vi "fgv_4610_visa.vi"(7 "cmd":T1, 8 "error in":errorcluster) -> (0 "error out":errorcluster)   [LabVIEW 2019]
uses:
  _ctrl/BP4610_cmd.ctl
  _ctrl/init-r-stop.ctl
  SubVIs/common/cmd_err.ctl
  _ctrl/rw.ctl
  Type def/SetNF_BP4610.ctl
  SubVIs/common/Glob_Ref.vi
panel:
  out "OverLoad":i32 caption="Query"
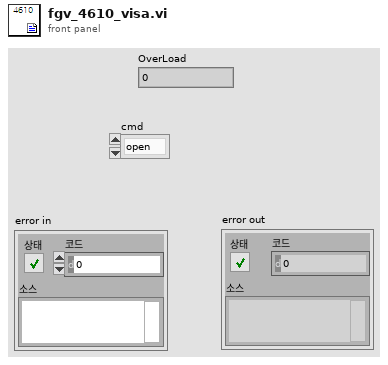
[diagram p1: front panel]
types:
  T1 = typedef "BP4610_cmd.ctl" = enum16{"open", "read", "set", "set_seq", "limit", "limit_seq", "output on", "output off", "close"}
  T2 = enum16{"DL950", "BP4610", "DSP1500", "cDAQ-AI", "cDAQ-AO", "cDAQ-DO"}
  T3 = typedef "init-r-stop.ctl" = enum16{"ini", "read", "stop"}
  T4 = typedef "cmd_err.ctl" = enum16{"close", "open", "default"}
  T5 = typedef "rw.ctl" = enum16{"read", "write"}
  T6 = typedef "SetNF_BP4610.ctl" = cluster{"Set":enum16{"Current", "Voltage", "FREQ/WAVE"}, "Operation mode":u16, "Voltage[Vp-p]":dbl, "Current[Ap-p]":dbl, "Voltage[V]":dbl, "Current[A]":dbl, "Frequency[Hz]":dbl, "Waveform":enum16{"Sine", "Square", "ARB 1", "ARB 2", "ARB 3", "ARB 4", "ARB 5", "ARB 6", "ARB 7", "ARB 8", "ARB 9", "ARB 10", "ARB 11", "ARB 12", "ARB 13", "ARB 14", "ARB 15", "ARB 16"}}
  T7 = typedef "BP4610_config.ctl" = cluster{"VISA":refnum<visa-resource-name>, "Limit-BP":cluster{"Set":enum16{"Current", "Voltage"}, "Voltage+[V]":dbl, "Current+[A]":dbl, "Voltage-[V]":dbl, "Current-[A]":dbl}, "SET BP":cluster{"Set":enum16{"Current", "Voltage", "FREQ/WAVE"}, "Operation mode":u16, "Voltage[Vp-p]":dbl, "Current[Ap-p]":dbl, "Voltage[V]":dbl, "Current[A]":dbl, "Frequency[Hz]":dbl, "Waveform":enum16{"Sine", "Square", "ARB 1", "ARB 2", "ARB 3", "ARB 4", "ARB 5", "ARB 6", "ARB 7", "ARB 8", "ARB 9", "ARB 10", "ARB 11", "ARB 12", "ARB 13", "ARB 14", "ARB 15", "ARB 16"}}}
  T8 = typedef "BP4610_return.ctl" = cluster{"DC voltage[V]":dbl, "DC current[A]":dbl}
  T9 = cluster{"Set":enum16{"Current", "Voltage", "FREQ/WAVE"}, "Operation mode":u16, "Voltage[Vp-p]":dbl, "Current[Ap-p]":dbl, "Voltage[V]":dbl, "Current[A]":dbl, "Frequency[Hz]":dbl, "Waveform":enum16{"Sine", "Square", "ARB 1", "ARB 2", "ARB 3", "ARB 4", "ARB 5", "ARB 6", "ARB 7", "ARB 8", "ARB 9", "ARB 10", "ARB 11", "ARB 12", "ARB 13", "ARB 14", "ARB 15", "ARB 16"}}
  T10 = typedef "cap_config.ctl" = cluster{"Test Mode":enum32{"6.3.2 저온 작동/방치 시험", "6.3.3 고온 작동/방치 시험", "6.3.4 온도 싸이클 시험", "6.3.6 온습도 싸이클 시험", "6.3.8 결로 시험", "6.3.9 빙결 시험", "ON/OFF 동작시험"}, "ON time[ms]":dbl, "OFF time[ms]":dbl, "1. 작동시간[분]":dbl, "2. 미작동시간[분]":dbl, "3. 작동시간[분]":dbl, "level[V]":dbl, "duty":dbl, "Freq":dbl, "Voltage+[V]":dbl, "Voltage-[V]":dbl, "Current+[A]":dbl, "Current-[A]":dbl, "출력전압[V]":dbl, "출력전류[A]":dbl, "OVP Level":dbl, "OCP Level":dbl, "Time Div":u16, "Record Len":i32, "방전 기준[V]":dbl, "Repeate (Each Ch)":u32, "Cycle[N]":u32, "ON/OFF 회 수[N]":dbl, "TrigPos[%]":dbl, "시험시간[분]":dbl}
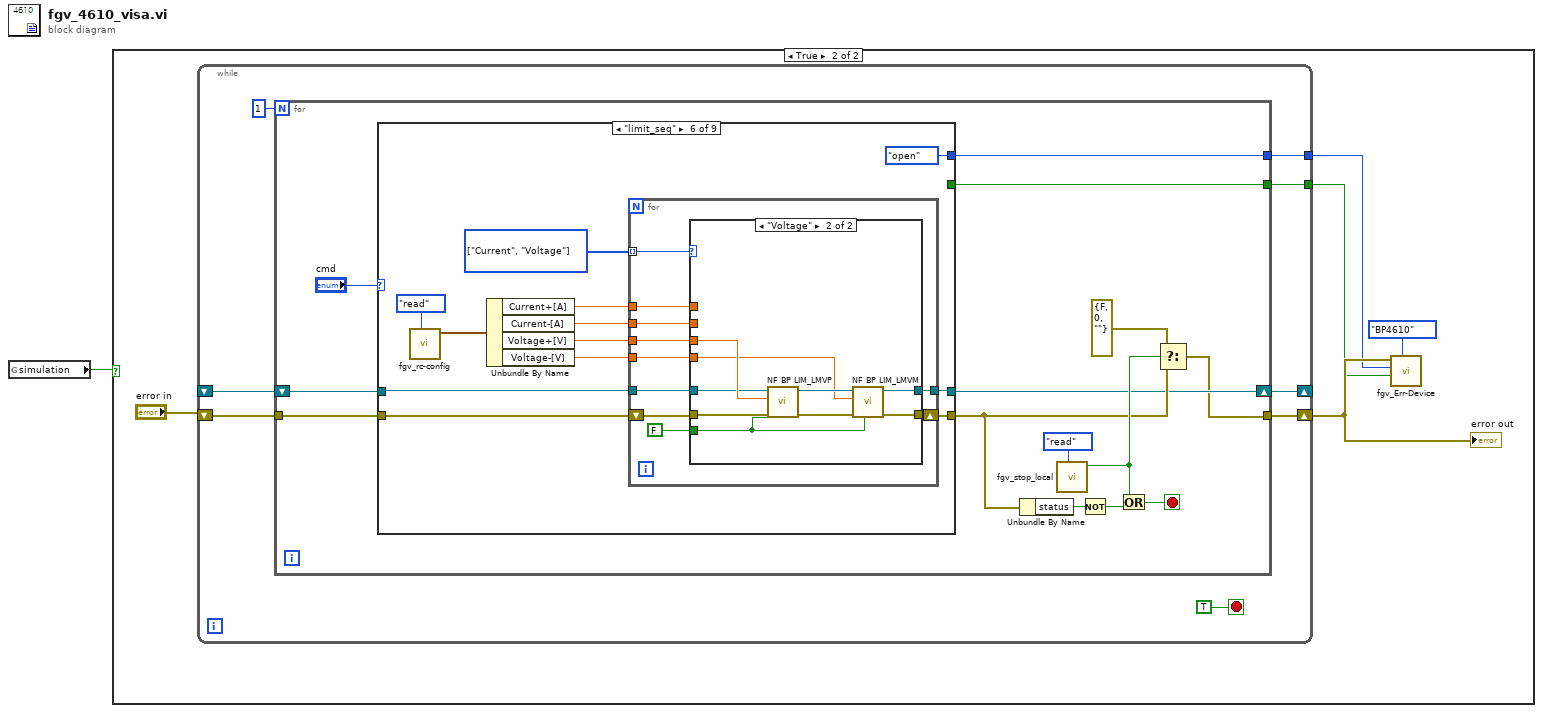
[diagram p0: block diagram]
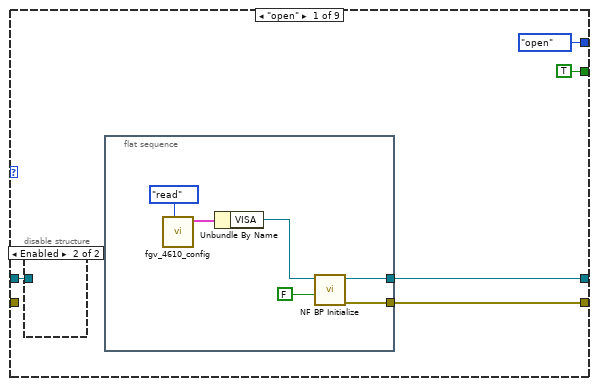
[diagram p3: hidden frame]
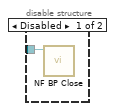
[diagram p4: hidden frame]
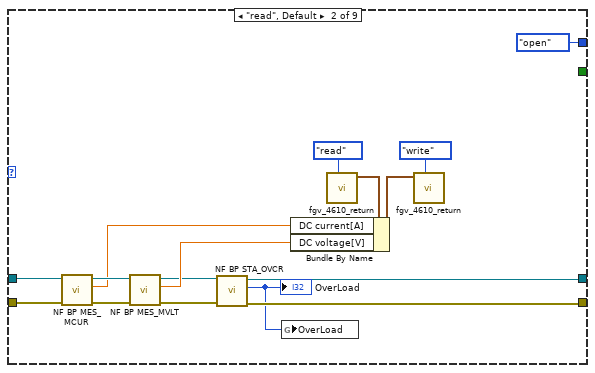
[diagram p5: hidden frame]
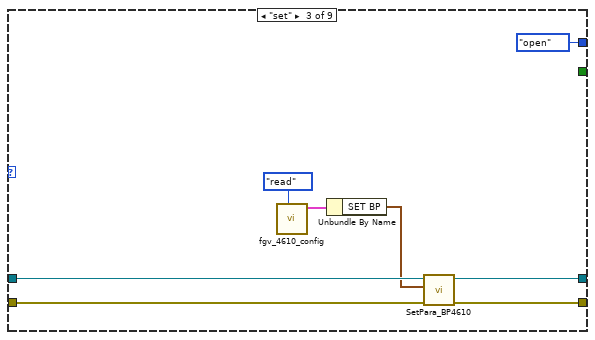
[diagram p6: hidden frame]
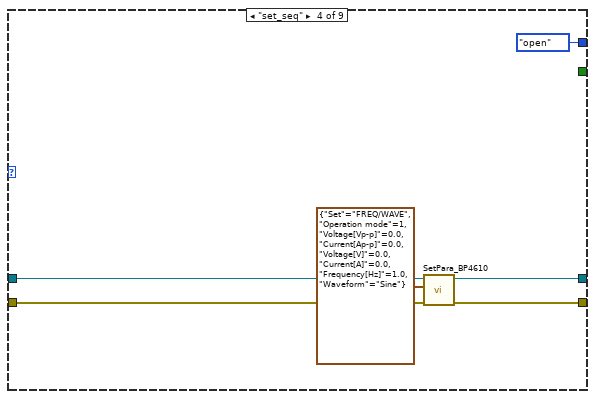
[diagram p7: hidden frame]
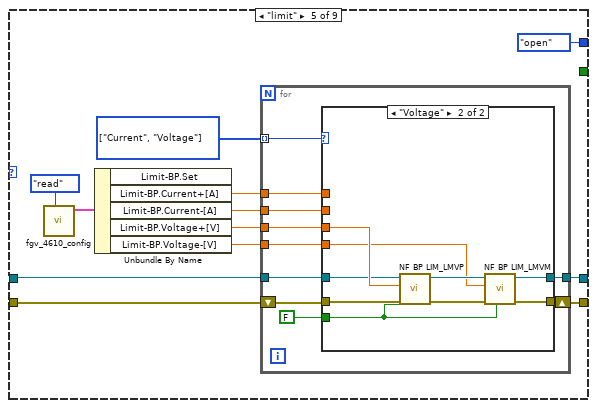
[diagram p8: hidden frame]
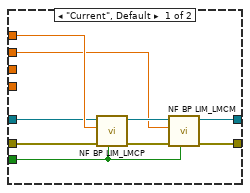
[diagram p9: hidden frame]
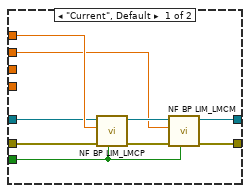
[diagram p10: hidden frame]
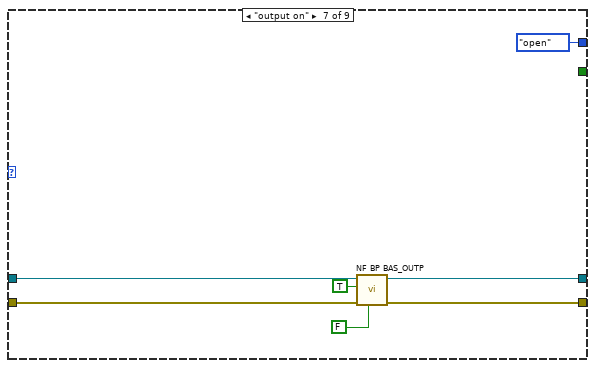
[diagram p11: hidden frame]
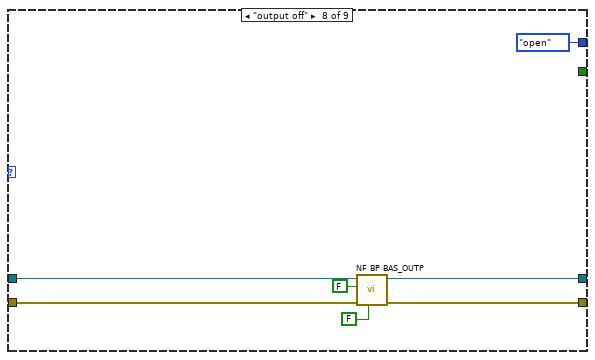
[diagram p12: hidden frame]
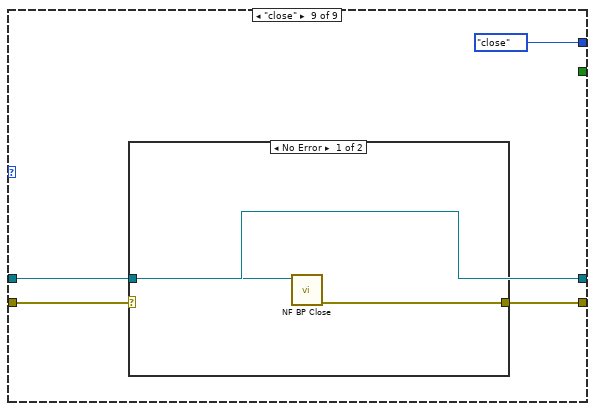
[diagram p13: hidden frame]
diagram:
  n1 = global read "Glob_Ref.vi" "simulation"() -> (w1:bool)
  n2 = case shown="True" w1 {
    frame False {
    }
    frame True {
      n3 = while {
        shift-right: [w11] -> _
        shift-left: _ -> [w13]
        shift-right: [w12] -> w5
        shift-left: "error in" -> [w9]
        tunnel: [w8] -> w4
        tunnel: [w7] -> w3
        stop <- TRUE stop-if-true
        n4 = for {
          N: 1 -> [_]
          tunnel: [w15] -> w12
          shift-right: [w16] -> w11
          shift-left: w13 -> [w27]
          tunnel: w9 -> [w19]
          tunnel: [w18] -> w8
          tunnel: [w17] -> w7
          stop <- w20 stop-if-true
          n5 = case shown="\"limit_seq\"" "cmd" {
            tunnel: [w33 w43 w64 w70 w80 w120 w153 w160 w166] -> w21
            tunnel: [w32 w44 w63 w69 w79 w119 w154 w161 w168] -> w16
            tunnel: w19 -> [_ w54 w61 w67 w81 w121 w155 w162 w167]
            tunnel: w27 -> [w31 w53 w62 w68 w82 w122 w156 w163 w168]
            tunnel: [cmd_err."open" ("cmd") cmd_err."open" ("cmd") cmd_err."open" ("cmd") cmd_err."open" ("cmd") cmd_err."open" ("cmd") cmd_err."open" ("cmd") cmd_err."open" ("cmd") cmd_err."open" ("cmd") cmd_err."close" ("cmd")] -> w18
            tunnel: [TRUE ("first?") _ _ _ _ _ _ _ _] -> w17
            frame "open" {
              n6 = disable-structure shown="Enabled" {
                disable-tunnel: w31 -> [w34 _]
                frame Disabled {
                  n7 = call <instrlib>:"NF BP Close.vi"("VISAsession"=w34) -> ()  [unwired: 10 in, 1 out]
                }
                frame Enabled {
                }
              }
              n8 = flat-sequence {
                tunnel: [w39] -> w33
                tunnel: [w38] -> w32
                frame #0 {
                  n9 = call "fgv_4610_config.vi"("cmd"=rw."read") -> ("BP4610 Config 2"=w36:T7)  [unwired: 9 in, 1 out]
                  n10 = Unbundle By Name(w36) -> ("VISA"=w35:refnum<visa-resource-name>)
                  n11 = call <instrlib>:"NF BP Initialize.vi"("Reset(T)"=FALSE ("Read"), "VISAsession"=w35) -> ("error out"=w39:errorcluster, "CopyVISAsession"=w38:refnum<visa-resource-name>)  [unwired: 7 in, 1 out]
                }
              }
            }
            frame "read", Default {
              n12 = call <instrlib>:"NF BP MES_MCUR.vi"("error in (no error)"=w54, "VISAsession"=w53) -> ("error out"=w56:errorcluster, "Query[A]"=w51:dbl, "CopyVISAsession"=w55:refnum<visa-resource-name>)  [unwired: 5 in, 2 out]
              n13 = call <instrlib>:"NF BP MES_MVLT.vi"("error in (no error)"=w56, "VISAsession"=w55) -> ("error out"=w45:errorcluster, "Query[V]"=w50:dbl, "CopyVISAsession"=w46:refnum<visa-resource-name>)  [unwired: 5 in, 2 out]
              n14 = call <instrlib>:"NF BP STA_OVCR.vi"("error in (no error)"=w45, "VISAsession"=w46) -> ("error out"=w43:errorcluster, "Query"=w42:i32, "CopyVISAsession"=w44:refnum<visa-resource-name>)  [unwired: 6 in, 1 out]
              "OverLoad" <- w42
              n15 = global write "Glob_Ref.vi" "OverLoad"(w42) -> ()
              n16 = call "fgv_4610_return.vi"("cmd"=rw."read") -> ("output 2"=w47:T8)  [unwired: 10 in]
              n17 = Bundle By Name(cluster=w47, "DC current[A]"=w51, "DC voltage[V]"=w50) -> (w49:T8)
              n18 = call "fgv_4610_return.vi"("cmd"=rw."write", "output"=w49) -> ()  [unwired: 9 in, 1 out]
            }
            frame "set" {
              n19 = call "fgv_4610_config.vi"("cmd"=rw."read") -> ("BP4610 Config 2"=w59:T7)  [unwired: 9 in, 1 out]
              n20 = Unbundle By Name(w59) -> ("SET BP"=w58:T9)
              n21 = call "SetPara_BP4610.vi"("error in"=w61, "SetBP"=w58, "VISA"=w62) -> ("error out"=w64:errorcluster, "VISA out"=w63:refnum<visa-resource-name>)  [unwired: 7 in]
            }
            frame "set_seq" {
              n22 = call "SetPara_BP4610.vi"("error in"=w67, "SetBP"=T6 {"Set"=enum."FREQ/WAVE", "Operation mode"=1, "Voltage[Vp-p]"=0.0, "Current[Ap-p]"=0.0, "Voltage[V]"=0.0, "Current[A]"=0.0, "Frequency[Hz]"=1.0, "Waveform"=enum."Sine"}, "VISA"=w68) -> ("error out"=w70:errorcluster, "VISA out"=w69:refnum<visa-resource-name>)  [unwired: 7 in]
            }
            frame "limit" {
              w72 = enum16{"Current", "Voltage"}[] [enum."Current", enum."Voltage"] items=["Current", "Voltage"]
              n23 = call "fgv_4610_config.vi"("cmd"=rw."read") -> ("BP4610 Config 2"=w77:T7)  [unwired: 9 in, 1 out]
              n24 = Unbundle By Name(w77) -> ("Limit-BP.Current+[A]"=w76:dbl, "Limit-BP.Current-[A]"=w75:dbl, "Limit-BP.Voltage+[V]"=w74:dbl, "Limit-BP.Voltage-[V]"=w73:dbl)  [unwired: 1 out]
              n25 = for {
                tunnel: w82 -> [w91]
                tunnel: [w88] -> w79
                tunnel: w76 -> [w87]
                tunnel: w75 -> [w86]
                tunnel: w74 -> [w85]
                tunnel: w73 -> [w84]
                shift-right: [w89] -> w80
                shift-left: w81 -> [w90]
                tunnel: w72 -> [w83] mode=indexing
                n26 = case shown="\"Voltage\"" w83 {
                  tunnel: w90 -> [w99 w110]
                  tunnel: [w101 w108] -> w89
                  tunnel: FALSE ("Read") -> [w98 w107]
                  tunnel: [w96 w105] -> w88
                  tunnel: w85 -> [_ w104]
                  tunnel: w84 -> [_ w103]
                  tunnel: w87 -> [w95 _]
                  tunnel: w86 -> [w94 _]
                  tunnel: w91 -> [w93 w102]
                  frame "Current", Default {
                    n27 = call <instrlib>:"NF BP LIM_LMCP.vi"("Read(F)"=w98, "error in (no error)"=w99, "Current[A]"=w95, "VISAsession"=w93) -> ("error out"=w100:errorcluster, "CopyVISAsession"=w97:refnum<visa-resource-name>)  [unwired: 4 in, 2 out]
                    n28 = call <instrlib>:"NF BP LIM_LMCM.vi"("Read(F)"=w98, "error in (no error)"=w100, "Current[A]"=w94, "VISAsession"=w97) -> ("error out"=w101:errorcluster, "CopyVISAsession"=w96:refnum<visa-resource-name>)  [unwired: 4 in, 2 out]
                  }
                  frame "Voltage" {
                    n29 = call <instrlib>:"NF BP LIM_LMVP.vi"("Read(F)"=w107, "error in (no error)"=w110, "Voltage[V]"=w104, "VISAsession"=w102) -> ("error out"=w109:errorcluster, "CopyVISAsession"=w106:refnum<visa-resource-name>)  [unwired: 4 in, 2 out]
                    n30 = call <instrlib>:"NF BP LIM_LMVM.vi"("Read(F)"=w107, "error in (no error)"=w109, "Voltage[V]"=w103, "VISAsession"=w106) -> ("error out"=w108:errorcluster, "CopyVISAsession"=w105:refnum<visa-resource-name>)  [unwired: 4 in, 2 out]
                  }
                }
              }
            }
            frame "limit_seq" {
              w114 = enum16{"Current", "Voltage"}[] [enum."Current", enum."Voltage"] items=["Current", "Voltage"]
              n31 = call "fgv_rc-config.vi"("cmd"=rw."read") -> ("Testconfig out"=w112:T10)  [unwired: 9 in, 1 out]
              n32 = Unbundle By Name(w112) -> ("Current+[A]"=w118:dbl, "Current-[A]"=w117:dbl, "Voltage+[V]"=w116:dbl, "Voltage-[V]"=w115:dbl)
              n33 = for {
                tunnel: w122 -> [w131]
                tunnel: [w128] -> w119
                tunnel: w118 -> [w127]
                tunnel: w117 -> [w126]
                tunnel: w116 -> [w125]
                tunnel: w115 -> [w124]
                shift-right: [w129] -> w120
                shift-left: w121 -> [w130]
                tunnel: w114 -> [w123] mode=indexing
                n34 = case shown="\"Voltage\"" w123 {
                  tunnel: w130 -> [w139 w150]
                  tunnel: [w141 w148] -> w129
                  tunnel: FALSE ("Read") -> [w138 w147]
                  tunnel: [w136 w145] -> w128
                  tunnel: w125 -> [_ w144]
                  tunnel: w124 -> [_ w143]
                  tunnel: w127 -> [w135 _]
                  tunnel: w126 -> [w134 _]
                  tunnel: w131 -> [w133 w142]
                  frame "Current", Default {
                    n35 = call <instrlib>:"NF BP LIM_LMCP.vi"("Read(F)"=w138, "error in (no error)"=w139, "Current[A]"=w135, "VISAsession"=w133) -> ("error out"=w140:errorcluster, "CopyVISAsession"=w137:refnum<visa-resource-name>)  [unwired: 4 in, 2 out]
                    n36 = call <instrlib>:"NF BP LIM_LMCM.vi"("Read(F)"=w138, "error in (no error)"=w140, "Current[A]"=w134, "VISAsession"=w137) -> ("error out"=w141:errorcluster, "CopyVISAsession"=w136:refnum<visa-resource-name>)  [unwired: 4 in, 2 out]
                  }
                  frame "Voltage" {
                    n37 = call <instrlib>:"NF BP LIM_LMVP.vi"("Read(F)"=w147, "error in (no error)"=w150, "Voltage[V]"=w144, "VISAsession"=w142) -> ("error out"=w149:errorcluster, "CopyVISAsession"=w146:refnum<visa-resource-name>)  [unwired: 4 in, 2 out]
                    n38 = call <instrlib>:"NF BP LIM_LMVM.vi"("Read(F)"=w147, "error in (no error)"=w149, "Voltage[V]"=w143, "VISAsession"=w146) -> ("error out"=w148:errorcluster, "CopyVISAsession"=w145:refnum<visa-resource-name>)  [unwired: 4 in, 2 out]
                  }
                }
              }
            }
            frame "output on" {
              n39 = call <instrlib>:"NF BP BAS_OUTP.vi"("Read(F)"=FALSE ("Read"), "error in (no error)"=w155, "State(OFF)"=TRUE, "VISAsession"=w156) -> ("error out"=w153:errorcluster, "CopyVISAsession"=w154:refnum<visa-resource-name>)  [unwired: 4 in, 2 out]
            }
            frame "output off" {
              n40 = call <instrlib>:"NF BP BAS_OUTP.vi"("Read(F)"=FALSE ("Read"), "error in (no error)"=w162, "State(OFF)"=FALSE, "VISAsession"=w163) -> ("error out"=w160:errorcluster, "CopyVISAsession"=w161:refnum<visa-resource-name>)  [unwired: 4 in, 2 out]
            }
            frame "close" {
              n41 = case shown="No Error" w167 {
                selector: w167 -> [_ w171]
                tunnel: w168 -> [w170 _]
                tunnel: [w169 w171] -> w166
                frame No Error {
                  n42 = call <instrlib>:"NF BP Close.vi"("VISAsession"=w170) -> ("error out"=w169:errorcluster)  [unwired: 10 in]
                }
                frame Error {
                }
              }
            }
          }
          n43 = Unbundle By Name(w21) -> ("status"=w24:bool)
          n44 = call "fgv_stop_local.vi"("cmd"=init-r-stop."read") -> ("stop"=w22:bool)  [unwired: 9 in, 1 out]
          n45 = Not(x=w24) -> (.not. x?=w23:bool)
          n46 = Or(x=w22, y=w23) -> (x .or. y?=w20:bool)
          n47 = Select(t=errorcluster {"status"=FALSE, "code"=0, "source"=""}, s=w22, f=w21) -> (s? t:f=w15:errorcluster)
        }
      }
      "error out" <- w5
      n48 = call "fgv_Err-Device.vi"("Err Sel"=T2."BP4610", "first?"=w3, "cmd"=w4, "error in"=w5) -> ()  [unwired: 8 in]
    }
  }
